vi "fibbomen.vi"() -> ()   [LabVIEW 2021]
panel:
  out "XY Graph":cluster{i32[], i32[]}(graph)
  out "fibo numbers":i32[](array[numeric])
  in  "Enter N":i32
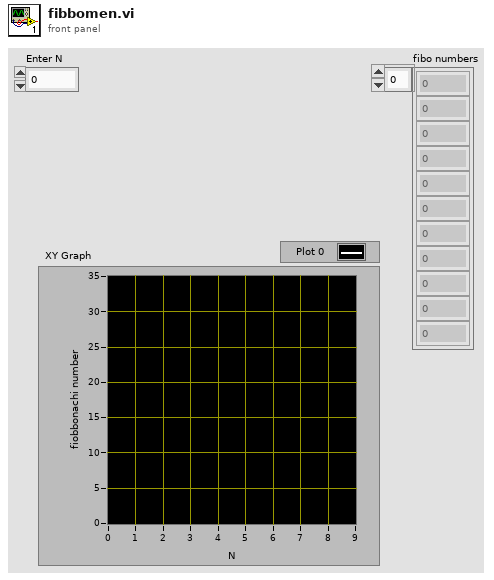
[diagram p1: front panel]
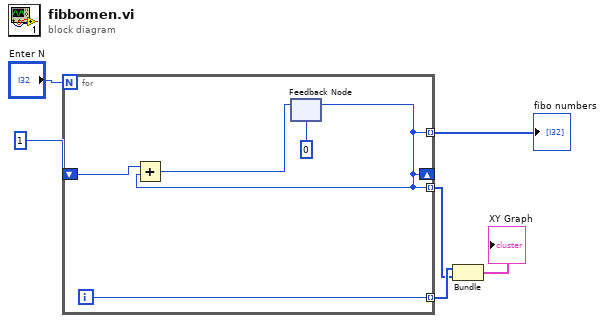
[diagram p0: block diagram]
diagram:
  n1 = for {
    N: "Enter N" -> [_]
    shift-right: [w7] -> _
    shift-left: 1 -> [w11]
    tunnel: [w7] -> w4 mode=indexing
    tunnel: [w8] -> w2 mode=indexing
    tunnel: [w7] -> w1 mode=indexing
    i -> [w8]
    n2 = feedback #1(0) -> (w7:i32)
    n3 = Add(x=w11, y=w7) -> (x+y=w10:i32)
    n4 = feedback-in #1(w10) -> ()
  }
  "fibo numbers" <- w4
  n5 = Bundle(w2, w1) -> (→"XY Graph":cluster{i32[], i32[]})  [unwired: 1 in]
